vi "Calibration-Frame2.vi"(10 "Mode in":T1, 11 "Results file output":path) -> (1 "data mode":enum16{"Take new data point", "Refit Curve"}(ring), 2 "Mode out":T1, 3 "Boolean":bool)   [LabVIEW 2015]
uses:
  Anemometry Sub Vis/Calibration/Calib_mode.ctl
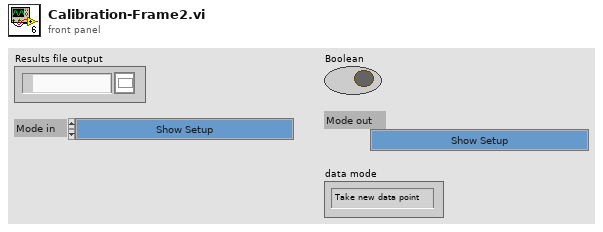
[diagram p1: front panel]
types:
  T1 = typedef "Calib_mode.ctl" = enum16{"Show Setup", "Take a New Calibration Point", "Refit Curve", "Setup Front Panel"}
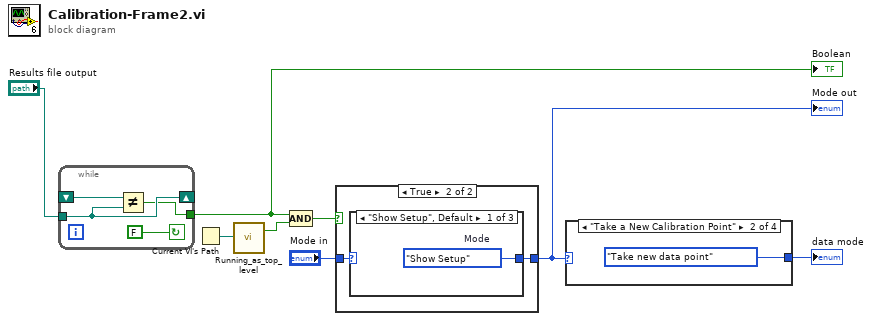
[diagram p0: block diagram]
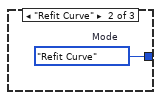
[diagram p3: hidden frame]
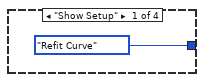
[diagram p5: hidden frame]
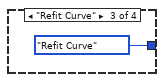
[diagram p6: hidden frame]
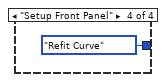
[diagram p7: hidden frame]
diagram:
  n1 = while {
    shift-right: [w11] -> _
    shift-left: _ -> [w12]
    tunnel: "Results file output" -> [w11]
    tunnel: [w10] -> w4
    stop <- FALSE continue-if-true
    n2 = Not Equal?(x=w12, y=w11) -> (x != y?=w10:bool)
  }
  "Boolean" <- w4
  n3 = Current VI's Path() -> (path=w2:path)
  n4 = call "Running_as_top_level.vi"("Vi path name"=w2) -> ("Top Level"=w8:bool)  [unwired: 1 out]
  n5 = Compound Arithmetic op=AND(w4, w8) -> (w5:bool)
  n6 = case shown="True" w5 {
    tunnel: "Mode in" -> [w13 w14]
    tunnel: [w13 w15] -> w7
    frame False {
    }
    frame True {
      n7 = case shown="\"Show Setup\", Default" w14 {
        selector: w14 -> [_ _ w18]
        tunnel: [w16 w17 w18] -> w15
        frame "Show Setup", Default {
          w16 = Calib_mode."Show Setup"  # Mode
        }
        frame "Refit Curve" {
          w17 = Calib_mode."Refit Curve"  # Mode
        }
        frame "Setup Front Panel" {
        }
      }
    }
  }
  "Mode out" <- w7
  n8 = case shown="\"Take a New Calibration Point\"" w7 {
    tunnel: [enum16{"Take new data point", "Refit Curve"}."Refit Curve" ("data mode") enum16{"Take new data point", "Refit Curve"}."Take new data point" ("data mode") enum16{"Take new data point", "Refit Curve"}."Refit Curve" ("data mode") enum16{"Take new data point", "Refit Curve"}."Refit Curve" ("data mode")] -> w1
    frame "Show Setup" {
    }
    frame "Take a New Calibration Point" {
    }
    frame "Refit Curve" {
    }
    frame "Setup Front Panel" {
    }
  }
  "data mode" <- w1
